vi "Generate calibration data listbox array .vi"(7 "Sr No.":i32[](array[numeric]), 8 "error in (no error)":errorcluster, 9 "Imaging Parameters":T2[](array[typedef]), 10 "Calibration data":T1[](array[typedef]), 11 "Imag ref. name":string[](array[string])) -> (0 "error out":errorcluster, 2 "LB data full":string[][](array[string]), 3 "LB data trunc":string[][](array[string]))   [LabVIEW 2020]
uses:
  TypeDefs/Current Imaging Parameters.ctl
  TypeDefs/Current Calibration Parameters.ctl
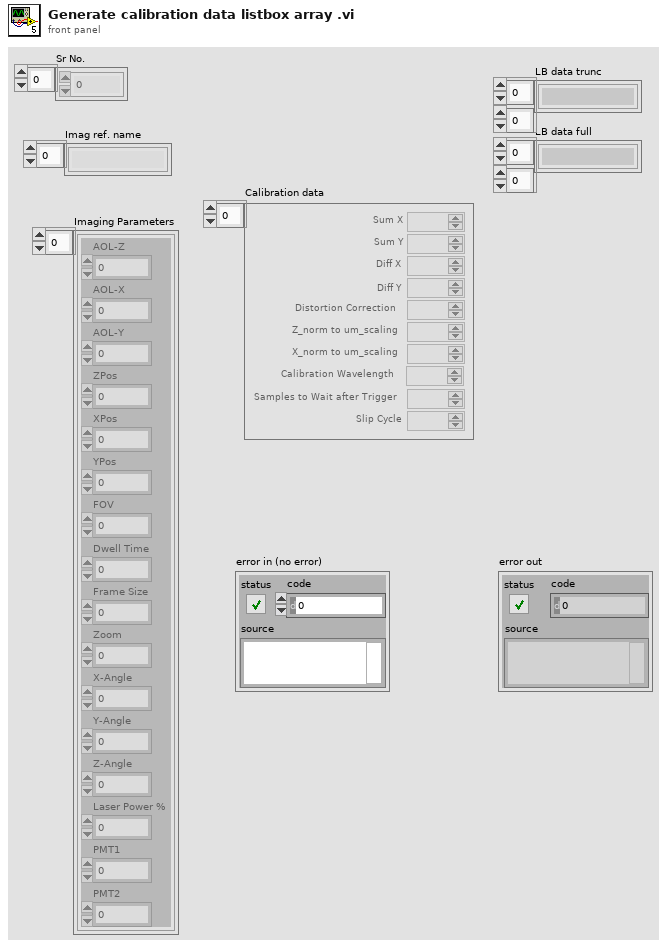
[diagram p1: front panel]
types:
  T1 = typedef "Current Calibration Parameters.ctl" = cluster{"Sum X":dbl, "Sum Y":dbl, "Diff X":dbl, "Diff Y":dbl, "Distortion Correction":dbl, "Z_norm to um_scaling":dbl, "X_norm to um_scaling":dbl, "Samples to Wait after Trigger":dbl, "Slip Cycle":dbl, "Calibration Wavelength":dbl}
  T2 = typedef "Current Imaging Parameters.ctl" = cluster{"AOL-Z":dbl, "AOL-X":dbl, "AOL-Y":dbl, "ZPos":dbl, "XPos":dbl, "YPos":dbl, "FOV":dbl, "Dwell Time":dbl, "Frame Size":dbl, "Zoom":dbl, "X-Angle":dbl, "Y-Angle":dbl, "Z-Angle":dbl, "Laser Power %":dbl, "PMT1":dbl, "PMT2":dbl}
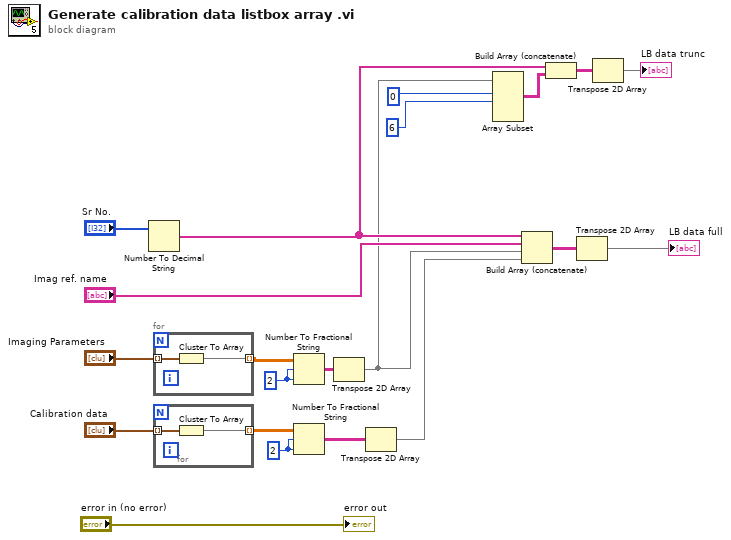
[diagram p0: block diagram]
diagram:
  w16 = i16 2 ("precision (6)")
  w18 = i16 2 ("precision (6)")
  n1 = Number To Decimal String(number="Sr No.") -> (decimal integer string=w11:string[])  [unwired: 1 in]
  n2 = for {
    tunnel: "Imaging Parameters" -> [w23] mode=indexing
    tunnel: [w22] -> w17 mode=indexing
    n3 = Cluster To Array(cluster=w23) -> (array=w22:dbl[])
  }
  n4 = for {
    tunnel: "Calibration data" -> [w25] mode=indexing
    tunnel: [w24] -> w15 mode=indexing
    n5 = Cluster To Array(cluster=w25) -> (array=w24:dbl[])
  }
  n6 = Number To Fractional String(number=w17, width (-)=w18, precision (6)=w18) -> (F-format string=w5:string[][])  [unwired: 1 in]
  n7 = Number To Fractional String(number=w15, width (-)=w16, precision (6)=w16) -> (F-format string=w7:string[][])  [unwired: 1 in]
  n8 = Transpose 2D Array(2D array=w5) -> (transposed array=w3:string[][])
  n9 = Transpose 2D Array(2D array=w7) -> (transposed array=w6:string[][])
  n10 = Array Subset(array=w3, index (row)=0 ("index"), length (row)=6 ("length")) -> (w10:string[][])  [unwired: 2 in]
  n11 = Build Array (concatenate)(w11, "Imag ref. name", w3, w6) -> (w14:string[][])
  n12 = Build Array (concatenate)(w11, w10) -> (w9:string[][])
  n13 = Transpose 2D Array(2D array=w14) -> (transposed array=→"LB data full":string[][])
  n14 = Transpose 2D Array(2D array=w9) -> (transposed array=→"LB data trunc":string[][])
  "error out" <- "error in (no error)"
